vi "Graph Sync.vi"(8 "error in (no error)":errorcluster, 11 "Control Ref Cluster":T1) -> (0 "error out":errorcluster, 1 "Plot Area Bounds":T3, 2 "Origin Coords":T4, 3 "Dup Control Ref Cluster":T1, 4 "Flip?":bool)   [LabVIEW 2020, in "2D Compass.lvclass"]
uses:
  <vilib>/Math Plots/2D Math Plots/2D Compass/2D Compass/2D Compass.lvclass
  <vilib>/Utility/miscctls.llb/LVPoint32TypeDef.ctl
  <vilib>/Math Plots/2D Math Plots/2D Plot/Action String/2DMathPlot Ctrl Act Cluster.ctl
  <vilib>/Math Plots/2D Math Plots/2D Plot/Action String/2DMathPlot State Class.ctl
  <vilib>/Math Plots/Plot Private Lib/NI_Math Plot Private Lib.lvlib
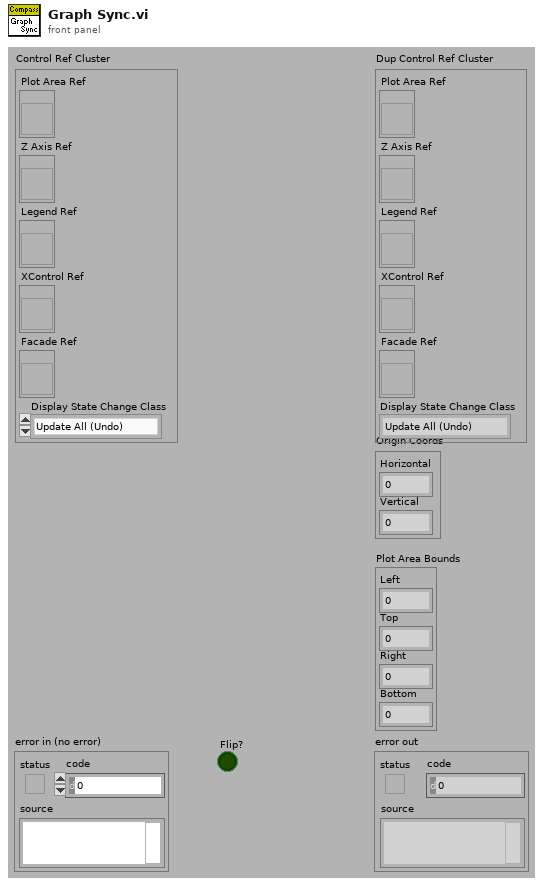
[diagram p1: front panel]
types:
  T1 = typedef "2DMathPlot Ctrl Act Cluster.ctl" = cluster{"Plot Area Ref":refnum<vi>, "Z Axis Ref":refnum<vi>, "Legend Ref":refnum<vi>, "XControl Ref":refnum<vi>, "Facade Ref":refnum<vi>, "Display State Change Class":T2}
  T2 = typedef "2DMathPlot State Class.ctl" = enum16{"Update All (Undo)", "Update General", "Update Appearance", "Update Format", "Update Scale", "Update Marker", "Update Cursor", "None"}
  T3 = cluster{"Left":i32, "Top":i32, "Right":i32, "Bottom":i32}
  T4 = typedef "LVPoint32TypeDef.ctl" = cluster{"Horizontal":i32, "Vertical":i32}
  T5 = typedef "LVRectTypeDef.ctl" = cluster{"Left":i16, "Top":i16, "Right":i16, "Bottom":i16}
  T6 = cluster{"left":i32, "top":i32, "right":i32, "bottom":i32}
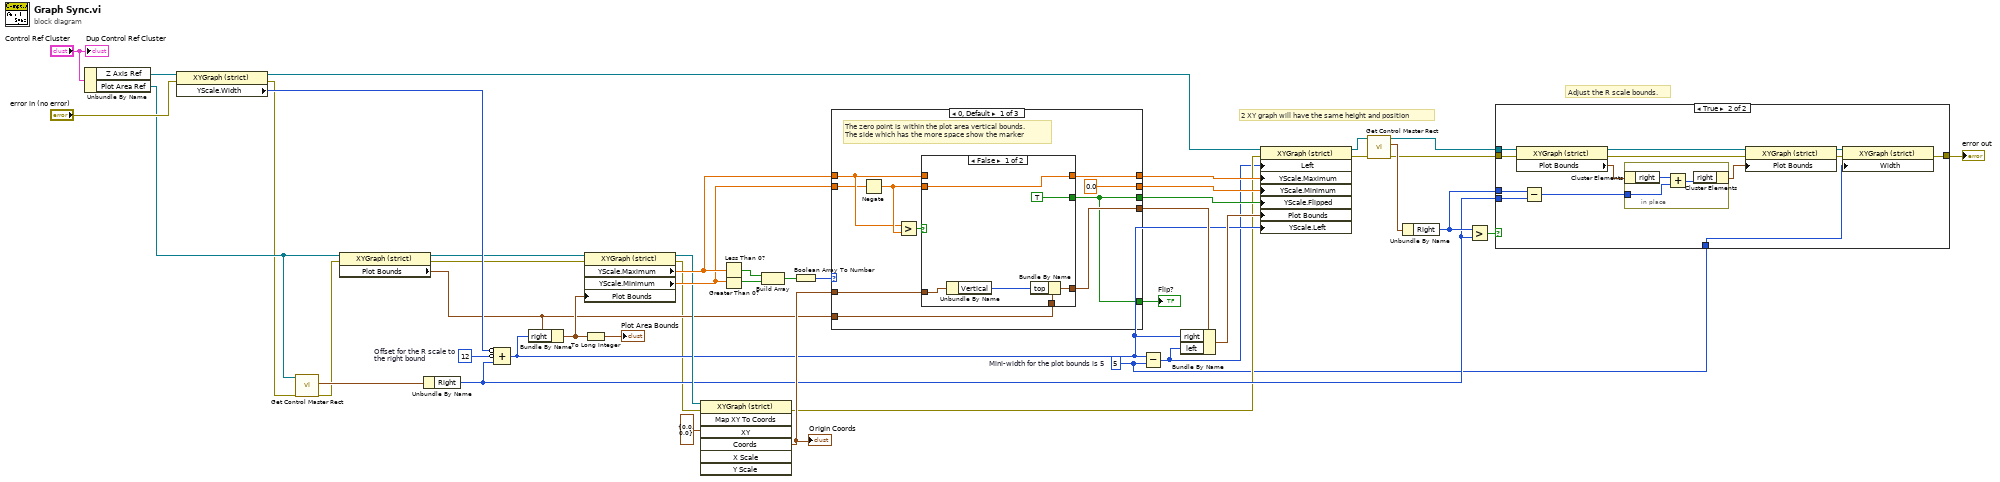
[diagram p0: block diagram]
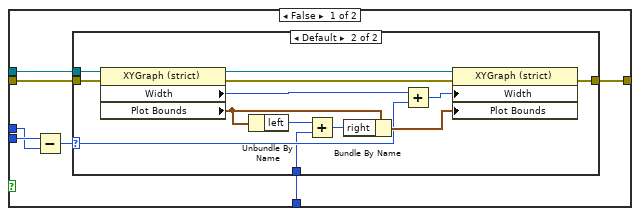
[diagram p2: hidden frame]
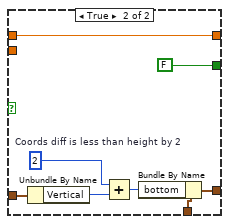
[diagram p4: hidden frame]
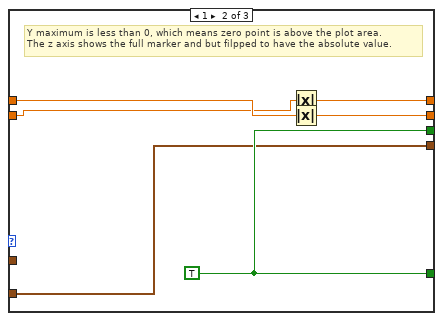
[diagram p5: hidden frame]
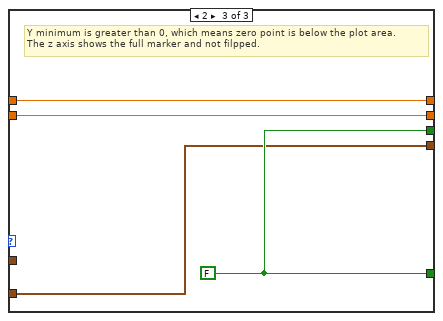
[diagram p6: hidden frame]
diagram:
  w29 = 12  # Offset for the R scale to the right bound
  w9 = u32 5  # Mini-width for the plot bounds is 5
  # "Adjust the R scale bounds."
  # "2 XY graph will have the same height and position"
  n1 = Unbundle By Name("Control Ref Cluster") -> ("Z Axis Ref"=w21:refnum<vi>, "Plot Area Ref"=w8:refnum<vi>)
  n2 = property class="XYGraph (strict)"(reference=w21, error in="error in (no error)") -> (reference out=w25:refnum<vi>, error out=w6:errorcluster, "YScale.Width"=w26:u32)
  n3 = call <vilib>:"Get Control Master Rect.vi"("error in (no error)"=w6, "reference"=w8) -> ("error out"=w5:errorcluster, "Master Bounds Rect"=w7:T5)  [unwired: 8 out]
  n4 = property class="XYGraph (strict)"(reference=w8, error in=w5) -> (reference out=w19:refnum<vi>, error out=w17:errorcluster, "Plot Bounds"=w15:T5)
  n5 = Unbundle By Name(w7) -> ("Right"=w13:i16)
  n6 = Compound Arithmetic op=ADD(invert w26, invert w29, w13) -> (w14:u32)
  n7 = Bundle By Name(cluster=w15, "right"=w14) -> (w20:T5)
  n8 = property class="XYGraph (strict)"(reference=w19, error in=w17, "Plot Bounds"=w20) -> (reference out=w16:refnum<vi>, error out=w12:errorcluster, "YScale.Maximum"=w33:dbl, "YScale.Minimum"=w32:dbl)
  n9 = To Long Integer(number=w20) -> (32bit integer=→"Plot Area Bounds":T6)
  n10 = invoke class="XYGraph (strict)" method="Map XY To Coords"(reference=w16, error in=w12, "XY"=cluster{"X":dbl, "Y":dbl} {"X"=0.0, "Y"=0.0}) -> (error out=w11:errorcluster, "Coords"=w42:T4)  [unwired: 4 in, 5 out]
  "Origin Coords" <- w42
  n11 = Less Than 0?(x=w33) -> (x < 0?=w40:bool)
  n12 = Greater Than 0?(x=w32) -> (x > 0?=w39:bool)
  n13 = Build Array(w40, w39) -> (w38:bool[])
  n14 = Boolean Array To Number(Boolean array=w38) -> (number=w37:u32)
  n15 = case shown="0, Default" w37 {
    tunnel: [w45 w69 w75] -> w41
    tunnel: w15 -> [w51 w68 w74]
    tunnel: w33 -> [w50 w73 w77]
    tunnel: w32 -> [w49 w72 w76]
    tunnel: [w48 w68 w74] -> w31
    tunnel: [w47 w71 w77] -> w36
    tunnel: [0.0 ("Y Scale.Range:Minimum") w70 w76] -> w35
    tunnel: [w45 w69 w75] -> w34
    tunnel: w42 -> [w44 _ _]
    frame 0, Default {
      # "The zero point is within the plot area vertical bounds. \nThe side which has the more space show the marker"
      n16 = Negate(x=w49) -> (-x=w52:dbl)
      n17 = Greater?(x=w50, y=w52) -> (0:w53:bool)
      n18 = case shown="False" w53 {
        tunnel: [TRUE ("Y Scale.Flipped") FALSE ("Y Scale.Flipped")] -> w45
        tunnel: w50 -> [_ w66]
        tunnel: [w58 w66] -> w47
        tunnel: w44 -> [w57 w62]
        tunnel: w51 -> [w56 w61]
        tunnel: [w55 w60] -> w48
        tunnel: w52 -> [w58 _]
        frame False {
          n19 = Unbundle By Name(w57) -> ("Vertical"=w54:i32)
          n20 = Bundle By Name(cluster=w56, "top"=w54) -> (w55:T5)
        }
        frame True {
          w63 = 2  # Coords diff is less than height by 2
          n21 = Unbundle By Name(w62) -> ("Vertical"=w65:i32)
          n22 = Add(x=w63, y=w65) -> (x+y=w64:i32)
          n23 = Bundle By Name(cluster=w61, "bottom"=w64) -> (w60:T5)
        }
      }
    }
    frame 1 {
      w69 = TRUE ("Y Scale.Flipped")
      # "Y maximum is less than 0, which means zero point is above the plot area.\nThe z axis shows the full marker and but filpped to have the absolute value."
      n24 = Absolute Value(x=w72) -> (abs(x)=w71:dbl)
      n25 = Absolute Value(x=w73) -> (abs(x)=w70:dbl)
    }
    frame 2 {
      w75 = FALSE ("Y Scale.Flipped")
      # "Y minimum is greater than 0, which means zero point is below the plot area.\nThe z axis shows the full marker and not filpped."
    }
  }
  "Flip?" <- w41
  n26 = Subtract(x=w14, y=w9) -> (x-y=w10:u32)
  n27 = Bundle By Name(cluster=w31, "right"=w14, "left"=w10) -> (w30:T5)
  n28 = property class="XYGraph (strict)"(reference=w25, error in=w11, "Left"=w10, "YScale.Maximum"=w36, "YScale.Minimum"=w35, "YScale.Flipped"=w34, "Plot Bounds"=w30, "YScale.Left"=w14) -> (reference out=w4:refnum<vi>, error out=w2:errorcluster)
  n29 = call <vilib>:"Get Control Master Rect.vi"("error in (no error)"=w2, "reference"=w4) -> ("error out"=w1:errorcluster, "Master Bounds Rect"=w3:T5)  [unwired: 8 out]
  n30 = Unbundle By Name(w3) -> ("Right"=w23:i16)
  n31 = Greater?(x=w23, y=w13) -> (0:w24:bool)
  n32 = case shown="True" w24 {
    tunnel: w4 -> [w84 w110]
    tunnel: w1 -> [w83 w109]
    tunnel: [w82 w101] -> w22
    tunnel: w13 -> [w81 w103]
    tunnel: w23 -> [w80 w104]
    tunnel: w9 -> [w78 w99]
    frame False {
      n33 = Subtract(x=w81, y=w80) -> (x-y=w79:i16)
      n34 = case shown="Default" w79 {
        selector: w79 -> [_ w87]
        tunnel: w84 -> [_ w97]
        tunnel: w83 -> [w85 w96]
        tunnel: [w85 w94] -> w82
        tunnel: w78 -> [_ w86]
        frame 0 {
        }
        frame Default {
          n35 = property class="XYGraph (strict)"(reference=w97, error in=w96) -> (reference out=w98:refnum<vi>, error out=w95:errorcluster, "Width"=w89:u32, "Plot Bounds"=w91:T5)
          n36 = Unbundle By Name(w91) -> ("left"=w93:i16)
          n37 = Add(x=w93, y=w86) -> (x+y=w90:u32)
          n38 = Bundle By Name(cluster=w91, "right"=w90) -> (w92:T5)
          n39 = Add(x=w89, y=w87) -> (x+y=w88:u32)
          n40 = property class="XYGraph (strict)"(reference=w98, error in=w95, "Width"=w88, "Plot Bounds"=w92) -> (error out=w94:errorcluster)  [unwired: 1 out]
        }
      }
    }
    frame True {
      n41 = property class="XYGraph (strict)"(reference=w110, error in=w109) -> (reference out=w108:refnum<vi>, error out=w107:errorcluster, "Plot Bounds"=w105:T5)
      n42 = Subtract(x=w104, y=w103) -> (x-y=w100:i16)
      n43 = in-place {
        in-place-border: w100 -> [w111]
        n44 = in-place-cluster #1(w105) -> ("right"=w113:i16)
        n45 = Add(x=w113, y=w111) -> (x+y=w112:i16)
        n46 = in-place-cluster #1("right"=w112) -> (w102:T5)
      }
      n47 = property class="XYGraph (strict)"(reference=w108, error in=w107, "Plot Bounds"=w102) -> (reference out=w106:refnum<vi>, error out=w101:errorcluster)
      n48 = property class="XYGraph (strict)"(reference=w106, "Width"=w99) -> ()  [unwired: 1 in, 2 out]
    }
  }
  "error out" <- w22
  "Dup Control Ref Cluster" <- "Control Ref Cluster"
